vi "WorkDisplay.vi"(3 "error in (no error)":errorcluster, 4 "idNumber":i32, 5 "Dll Path":path) -> (0 "error out":errorcluster)   [LabVIEW 2012]
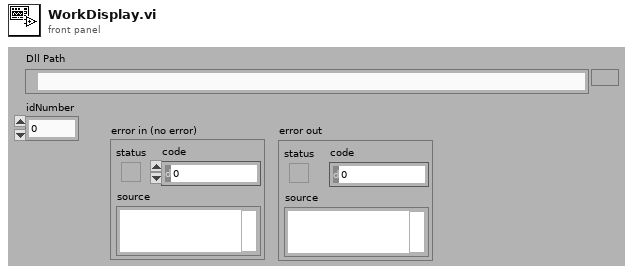
[diagram p1: front panel]
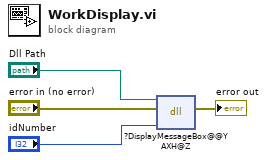
[diagram p0: block diagram]
diagram:
  n1 = dll-call lib="ThreadDll.dll" fn="?DisplayMessageBox@@YAXH@Z"(path in="Dll Path", error in="error in (no error)", "idNumber"="idNumber") -> (error out=→"error out":errorcluster)  [unwired: 3 in, 1 out]
